vi "Cleanup Session.vi"(8 "error in":errorcluster, 11 "Plugin in":refnum<class "AutomotiveDataSimulator.lvclass">) -> (0 "error out":errorcluster, 3 "Plugin out":refnum<class "AutomotiveDataSimulator.lvclass">)   [LabVIEW 2020, in "AutomotiveDataSimulator.lvlib" / "AutomotiveDataSimulator.lvclass"]
uses:
  AutomotiveDataSimulator.lvclass
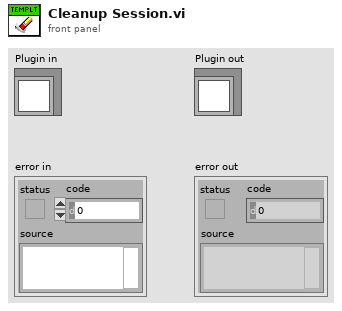
[diagram p1: front panel]
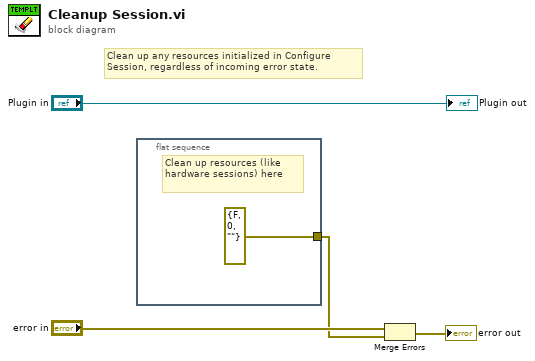
[diagram p0: block diagram]
diagram:
  # "Clean up any resources initialized in Configure Session, regardless of incoming error state."
  n1 = flat-sequence {
    tunnel: [errorcluster {"status"=FALSE, "code"=0, "source"=""} ("error in")] -> w1
    frame #0 {
      # "Clean up resources (like hardware sessions) here"
    }
  }
  n2 = Merge Errors("error in", w1) -> (→"error out":errorcluster)
  "Plugin out" <- "Plugin in"
